vi "Processing loop.vi"(8 "error in":errorcluster, 9 "Signal":refnum<vi>, 10 "Notify":refnum<notifier>, 11 "Processing Queue":refnum<queue>) -> (0 "error out":errorcluster)   [LabVIEW 2016]
uses:
  Queue Message Handler/Message Cluster.ctl
  <vilib>/addons/Biomedical/Biosignal Measurements/ECG/HRV analysis/subVIs/hrv statistics measures.ctl
  Control/Settings.ctl
  Control/port config.ctl
  <vilib>/LabVIEW Interface for Arduino/Type Defs/Board Type.ctl
  <vilib>/addons/Biomedical/Biosignal Measurements/Biosignal Preprocessing/subVIs/bmt_Rate Extractor_peak_valley.ctl
  <vilib>/measure/madcrms.llb/Basic Averaged DC-RMS for 1 Chan.vi
  <vilib>/measure/macond.llb/IIR Filter for 1 Chan.vi
  <vilib>/measure/matone.llb/Extract Single Tone Information 1 Chan.vi
  Queue Message Handler/Message Queue.lvlib
  <vilib>/LabVIEW Interface for Arduino/LabVIEW Interface for Arduino.lvlib
  <vilib>/measure/NI_MAPro.lvlib
  <vilib>/addons/Biomedical/NI_BMTK_Measurements.lvlib
panel:
  out "max value":dbl
  out "BPM":dbl
  out "Waveform Graph":waveform(dbl)(graph)
  out "detected frequency":dbl format="%.2p"
  out "statistics measurements":T1 {"RR mean" format="%#_4f"; "RR std" format="%#_4f"; "HR mean" format="%#_4f"; "HR std" format="%#_4f"; "RMSSD" format="%#_4f"}
  out "x-y":dbl
  out "Waveform Chart":dbl[](graph)
  in  "IIR bandpass":T2={"Topology"=enum."Butterworth", "Type"=enum."Bandpass", "Order"=2, "Lower Fc"=1.0, "Upper Fc"=5.0, "PB Ripple"=1.0, "SB Attenuation"=60.0} {"PB Ripple" format="%0.2f"; "SB Attenuation" format="%0.2f"; "Lower Fc" format="%0.2p"; "Upper Fc" format="%0.2p"}
  in  "IIR filter lowpass":T2={"Topology"=enum."Butterworth", "Type"=enum."Lowpass", "Order"=2, "Lower Fc"=15.0, "Upper Fc"=200.0, "PB Ripple"=1.0, "SB Attenuation"=60.0} {"PB Ripple" format="%0.2f"; "SB Attenuation" format="%0.2f"; "Lower Fc" format="%0.2p"; "Upper Fc" format="%0.2p"}
  in  "IIR filter highpass":T2={"Topology"=enum."Butterworth", "Type"=enum."Highpass", "Order"=2, "Lower Fc"=0.05, "Upper Fc"=200.0, "PB Ripple"=1.0, "SB Attenuation"=60.0} {"PB Ripple" format="%0.2f"; "SB Attenuation" format="%0.2f"; "Lower Fc" format="%0.2p"; "Upper Fc" format="%0.2p"}
  out "dt":dbl=0.005
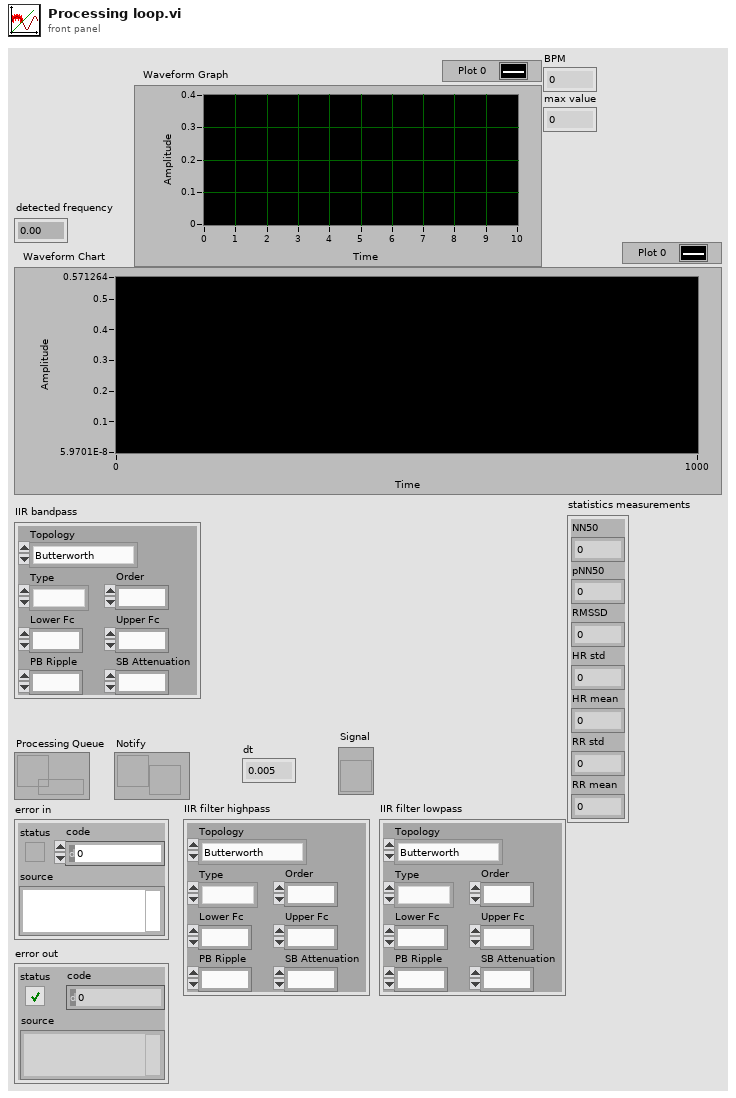
[diagram p1: front panel]
types:
  T1 = typedef "NI_BMTK_Measurements.lvlib/hrv statistics measures.ctl" = cluster{"NN50":i32, "pNN50":dbl, "RMSSD":dbl, "HR std":dbl, "HR mean":dbl, "RR std ":dbl, "RR mean":dbl}
  T2 = cluster{"Topology":enum16{"Off", "Butterworth", "Chebyshev", "Inverse Chebyshev", "Elliptic", "Bessel"}, "Type":enum16{"Lowpass", "Highpass", "Bandpass", "Bandstop"}, "Order":i32, "Lower Fc":dbl, "Upper Fc":dbl, "PB Ripple":dbl, "SB Attenuation":dbl}
  T3 = typedef "Settings.ctl" = cluster{"Port":T4, "Sample Rate (HZ)":u16, "Samples to Read":u16, "Input Pin":u8, "File path saved":path}
  T4 = typedef "port config.ctl" = cluster{"Port Name":refnum<visa-resource-name>, "Board Type":T5, "Baud Rate":u32}
  T5 = typedef "LabVIEW Interface for Arduino.lvlib/Board Type.ctl" = enum16{"Uno", "Dimuelanove w/Atmega 328", "Mega 2560"}
  T6 = typedef "NI_BMTK_Measurements.lvlib/bmt_Rate Extractor_peak_valley.ctl" = u16
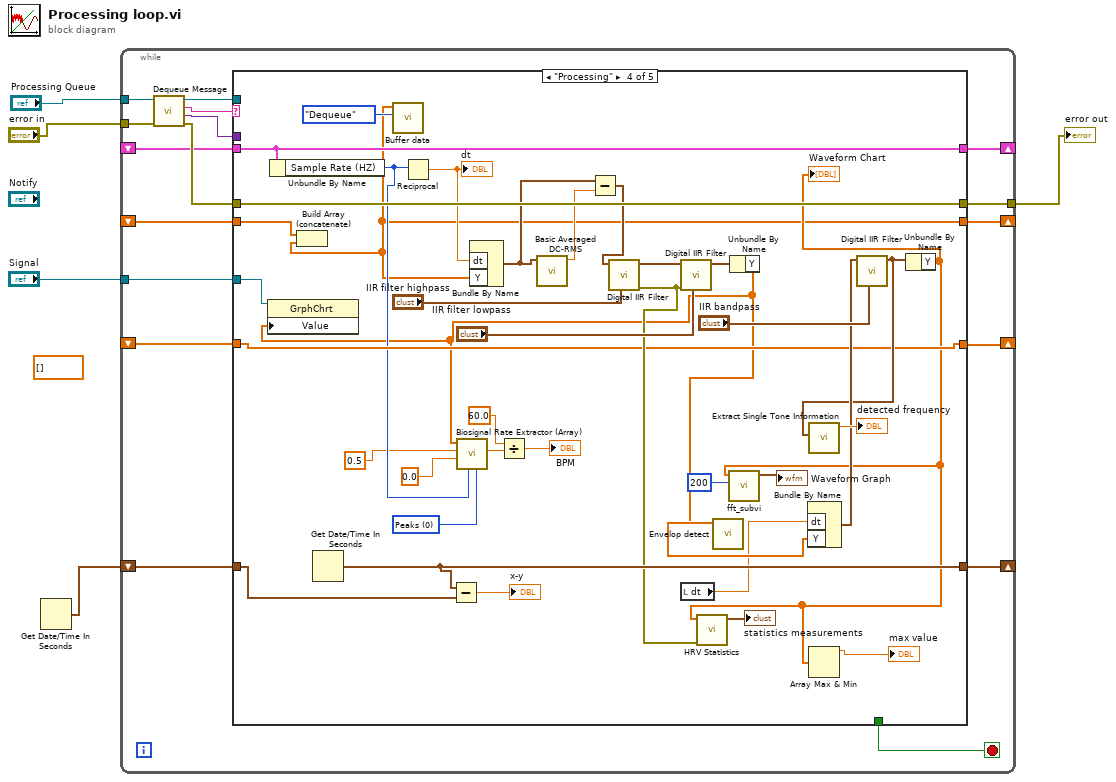
[diagram p0: block diagram]
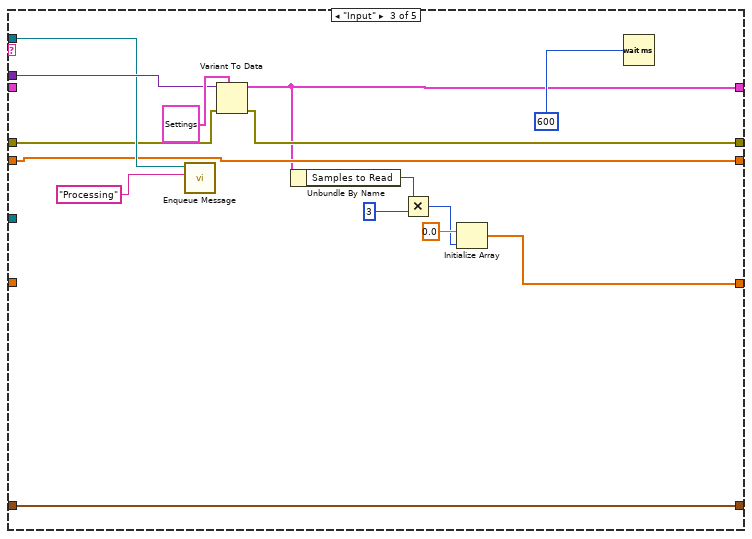
[diagram p4: hidden frame]
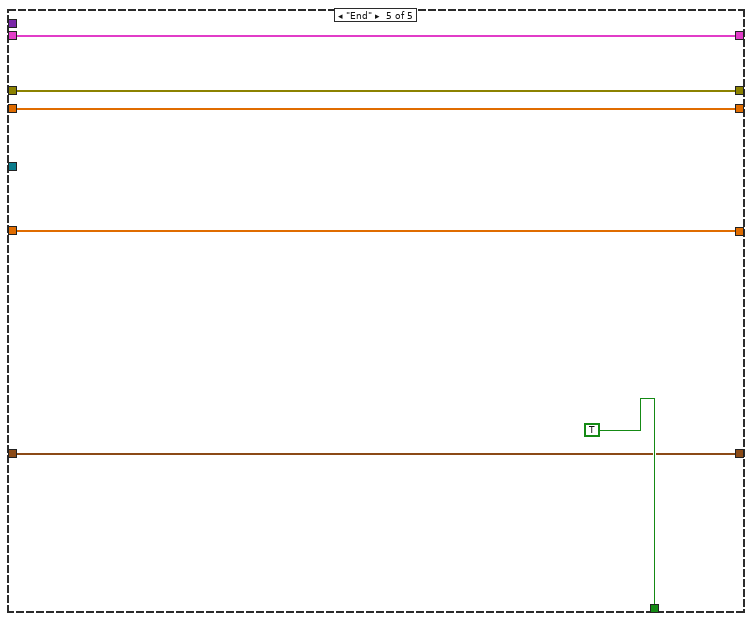
[diagram p5: hidden frame]
diagram:
  (unwired) dbl[] [] ("Y")
  n1 = Get Date/Time In Seconds() -> (seconds since 1Jan1904=w1:timestamp)
  n2 = while {
    tunnel: "Processing Queue" -> [w22]
    tunnel: "error in" -> [w21]
    tunnel: [w17] -> w3
    shift-right: [w15] -> _
    shift-left: _ -> [w14]
    shift-right: [w12] -> _
    shift-left: _ -> [w11]
    tunnel: "Signal" -> [w10]
    shift-right: [w9] -> _
    shift-left: w1 -> [w8]
    shift-right: [w7] -> _
    shift-left: _ -> [w6]
    stop <- w19 stop-if-true
    n3 = call "Dequeue Message.vi"("error in (no error)"=w21, "Message Queue"=w22) -> ("error out"=w18:errorcluster, "Message Data"=w16:variant, "Message"=w20:string, "dup Message Queue"=w13:refnum<queue>)  [unwired: 6 in]
    n4 = case shown="\"Processing\"" w20 {
      tunnel: [_ _ _ _ TRUE] -> w19
      tunnel: w18 -> [w27 w32 w42 w85 w90]
      tunnel: [w27 w32 w45 w85 w90] -> w17
      tunnel: w16 -> [_ _ w46 _ _]
      tunnel: [w26 w31 w37 w84 w89] -> w15
      tunnel: w14 -> [w26 w31 _ w84 w89]
      tunnel: w13 -> [_ _ w44 _ _]
      tunnel: [w25 w30 w41 w49 w88] -> w12
      tunnel: w11 -> [w25 w30 w41 w59 w88]
      tunnel: w10 -> [_ _ _ w78 _]
      tunnel: [w24 w29 w39 w73 w87] -> w9
      tunnel: w8 -> [w24 w29 w39 w72 w87]
      tunnel: [w23 w28 w33 w60 w86] -> w7
      tunnel: w6 -> [w23 w28 _ w60 w86]
      frame "False", Default {
      }
      frame "initial" {
      }
      frame "Input" {
        n5 = call "Enqueue Message.vi"("Message"="Processing", "Message Queue"=w44) -> ()  [unwired: 8 in, 2 out]
        n6 = Variant To Data(error in=w42, type=T3 {"Port"={"Port Name"="", "Board Type"=enum."Uno", "Baud Rate"=115200}, "Sample Rate (HZ)"=100, "Samples to Read"=50, "Input Pin"=0, "File path saved"=path ""} ("Settings out"), Variant=w46) -> (data=w37:T3, error out=w45:errorcluster)
        n7 = Unbundle By Name(w37) -> ("Samples to Read"=w36:u16)
        n8 = Multiply(x=w36, y=u16 3) -> (x*y=w34:u16)
        n9 = Initialize Array(0.0 ("element"), w34) -> (w33:dbl[])
        n10 = Wait (ms)(milliseconds to wait=u32 600) -> ()  [unwired: 1 out]
      }
      frame "Processing" {
        w54 = T6 0 items=["Peaks", "Valleys"] ("peaks/valleys")
        n11 = Unbundle By Name(w84) -> ("Sample Rate (HZ)"=w53:u16)
        n12 = Get Date/Time In Seconds() -> (seconds since 1Jan1904=w73:timestamp)
        n13 = call "Buffer data.vi"("Command"=enum16{"Create", "Enqueue", "Dequeue", "Clear"}."Dequeue") -> ("Data out"=w49:dbl[])  [unwired: 9 in, 1 out]
        n14 = Build Array (concatenate)(w59, w49) -> ()  [unwired: 1 out]
        n15 = Reciprocal(x=w53) -> (1/x=w82:dbl)
        "dt" <- w82
        n16 = Subtract(x=w73, y=w72) -> (x-y=→"x-y":dbl)
        n17 = Bundle By Name("dt"=w82, "Y"=w49) -> (w76:waveform(dbl))  [unwired: 1 in]
        n18 = call-poly <vilib>:"Basic Averaged DC-RMS.vi"("signal in"=w76) -> ("DC value"=w77:dbl)  [unwired: 7 in, 3 out]
        n19 = Subtract(x=w76, y=w77) -> (x-y=w75:waveform(dbl))
        n20 = call-poly <vilib>:"Digital IIR Filter.vi"("IIR filter specifications"="IIR filter highpass", "signal in"=w75) -> ("error out"=w69:errorcluster, "signal out"=w80:waveform(dbl))  [unwired: 7 in, 1 out]
        n21 = call-poly <vilib>:"Digital IIR Filter.vi"("IIR filter specifications"="IIR filter lowpass", "error in (no error)"=w69, "signal in"=w80) -> ("signal out"=w67:waveform(dbl))  [unwired: 6 in, 2 out]
        n22 = local read "dt"() -> (w64:dbl)
        n23 = Unbundle By Name(w67) -> ("Y"=w48:dbl[])
        n24 = property class="GrphChrt"(reference=w78, "Value"=w48) -> ()  [unwired: 1 in, 2 out]
        n25 = call <vilib>:"Biosignal Rate Extractor (Array).vi"("peaks/valleys"=w54, "sampling rate"=w53, "low threshold"=0.0, "high threshold"=0.5, "biosignal"=w48) -> ("mean cycle time"=w57:dbl)  [unwired: 4 in, 2 out]
        n26 = Divide(x=60.0, y=w57) -> (x/y=→"BPM":dbl)
        n27 = call "Envelop detect.vi"("Data in"=w48) -> ("Envelop"=w65:dbl[])  [unwired: 9 in, 1 out]
        n28 = Bundle By Name("dt"=w64, "Y"=w65) -> (w63:waveform(dbl))  [unwired: 1 in]
        n29 = call-poly <vilib>:"Digital IIR Filter.vi"("IIR filter specifications"="IIR bandpass", "signal in"=w63) -> ("signal out"=w62:waveform(dbl))  [unwired: 7 in, 2 out]
        n30 = call-poly <vilib>:"Extract Single Tone Information.vi"("export mode"=w62) -> ("detected frequency"=→"detected frequency":dbl)  [unwired: 5 in, 5 out]
        n31 = Unbundle By Name(w62) -> ("Y"=w52:dbl[])
        "Waveform Chart" <- w52
        n32 = call <vilib>:"HRV Statistics.vi"("error in (no error)"=w69, "raw RR"=w52) -> ("statistics measurements"=→"statistics measurements":T1)  [unwired: 8 in, 1 out]
        n33 = call "fft_subvi.vi"("Fs"=200, "Array"=w52) -> ("Waveform Graph"=→"Waveform Graph":waveform(dbl))  [unwired: 9 in]
        n34 = Array Max & Min(array=w52) -> (max value=→"max value":dbl)  [unwired: 3 out]
      }
      frame "End" {
      }
    }
  }
  "error out" <- w3
